vi "Lang Set Path.vi"(8 "error in (no error)":errorcluster, 10 "Path":T1, 11 "Configuration Window in":refnum<class "Configuration Window.lvclass">) -> (0 "error out":errorcluster, 3 "Configuration Window out":refnum<class "Configuration Window.lvclass">)   [LabVIEW 2018, in "Configuration Window.lvlib" / "Configuration Window.lvclass"]
uses:
  Configuration Window.lvclass
  Framework/Framework/Const Lang CfgWnd Path.ctl
  Framework/Framework/Const Lang Property.ctl
  Configuration Window.lvclass/Configuration Window.ctl
  Framework/Framework/Framework.lvclass
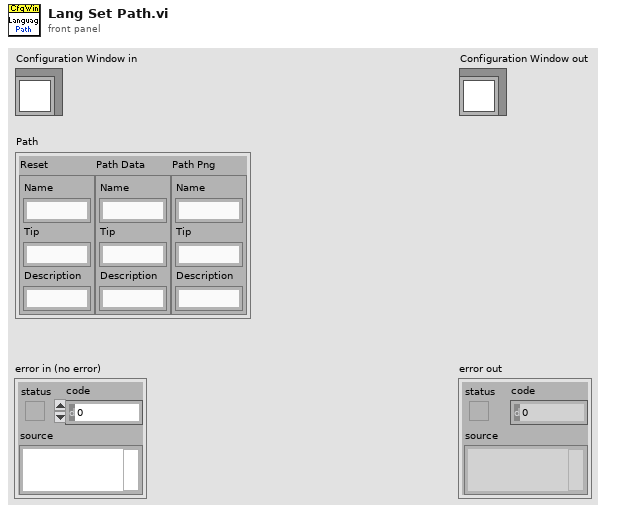
[diagram p1: front panel]
types:
  T1 = typedef "Framework.lvlib/Framework.lvclass/Const Lang CfgWnd Path.ctl" = cluster{"Reset":T2, "Path Data":T2, "Path Png":T2}
  T2 = typedef "Framework.lvlib/Framework.lvclass/Const Lang Property.ctl" = cluster{"Name":string, "Tip":string, "Description":string}
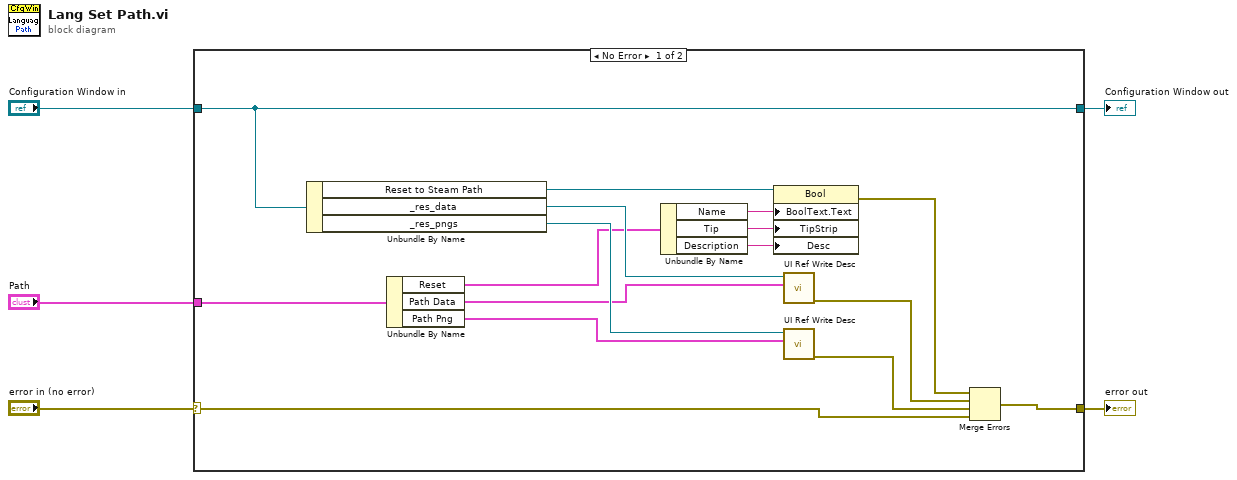
[diagram p0: block diagram]
diagram:
  n1 = case shown="No Error" "error in (no error)" {
    selector: "error in (no error)" -> [w6 w23]
    tunnel: [w19 w23] -> w4
    tunnel: [w21 w22] -> w2
    tunnel: "Configuration Window in" -> [w21 w22]
    tunnel: "Path" -> [w16 _]
    frame No Error {
      n2 = Unbundle By Name(w21) -> ("Reset to Steam Path"=w13:refnum<vi>, "_res_data"=w18:refnum<vi>, "_res_pngs"=w17:refnum<vi>)
      n3 = Unbundle By Name(w16) -> ("Reset"=w12:T2, "Path Data"=w15:T2, "Path Png"=w14:T2)
      n4 = Unbundle By Name(w12) -> ("Name"=w11:string, "Tip"=w10:string, "Description"=w9:string)
      n5 = property class="Bool"(reference=w13, "BoolText.Text"=w11, "TipStrip"=w10, "Desc"=w9) -> (error out=w7:errorcluster)  [unwired: 1 in, 1 out]
      n6 = call "UI Ref Write Desc.vi"("UI Property"=w15, "UI Ref"=w18) -> ("error out"=w20:errorcluster)  [unwired: 9 in]
      n7 = call "UI Ref Write Desc.vi"("UI Property"=w14, "UI Ref"=w17) -> ("error out"=w8:errorcluster)  [unwired: 9 in]
      n8 = Merge Errors(w7, w20, w8, w6) -> (w19:errorcluster)
    }
    frame Error {
    }
  }
  "error out" <- w4
  "Configuration Window out" <- w2
